vi "Dial Station Modem.vi"(8 "error in (no error)":errorcluster, 11 "Data Cluster in":T1={"Data Display"="", "FP Control Refs"={"Connect to Station Ref"=refnum, "Download Ref"=refnum, "Exit Button Ref"=refnum, "Start Date Refnum"=refnum, "End Date Refnum"=refnum, "Path"=refnum, "COM Port"="", "IP or Phone Ref"=refnum, "TCPIP ID"=refnum, "Reboot Refnum"=refnum, "Datafile Refnum"=refnum}, "FP Indicator Refs"={"Connected Refnum"=refnum, "Data Display Ref"=refnum, "Station ID Ref"=refnum}, "User Events"={"Stop"=refnum, "Update Display"=refnum}, "Message Queues"={"UI"=refnum, "ACQUISITION"=refnum, "PROCESSING"=refnum, "LOGGING"=refnum}, "IS IP?"=FALSE, "Downloading?"=FALSE, "DCP Version"=enum."XPert2", "Processing Loop State"=enum."Get Station  ID", "Username"=refnum, "Password"=refnum}) -> (0 "error out (no error)":errorcluster, 3 "Data Cluster out":T1={"Data Display"="", "FP Control Refs"={"Connect to Station Ref"=refnum, "Download Ref"=refnum, "Exit Button Ref"=refnum, "Start Date Refnum"=refnum, "End Date Refnum"=refnum, "Path"=refnum, "COM Port"="", "IP or Phone Ref"=refnum, "TCPIP ID"=refnum, "Reboot Refnum"=refnum, "Datafile Refnum"=refnum}, "FP Indicator Refs"={"Connected Refnum"=refnum, "Data Display Ref"=refnum, "Station ID Ref"=refnum}, "User Events"={"Stop"=refnum, "Update Display"=refnum}, "Message Queues"={"UI"=refnum, "ACQUISITION"=refnum, "PROCESSING"=refnum, "LOGGING"=refnum}, "IS IP?"=FALSE, "Downloading?"=FALSE, "DCP Version"=enum."XPert2", "Processing Loop State"=enum."Get Station  ID", "Username"=refnum, "Password"=refnum})   [LabVIEW 2018]
uses:
  controls/GLDL UI Data.ctl
  controls/Disconnect Control.ctl
  controls/Download Control.ctl
  controls/Exit Control.ctl
  controls/Date Control.ctl
  controls/IP Phone Number Control.ctl
  controls/Reboot Control.ctl
  controls/Connected Indicator.ctl
  controls/Output Indicator.ctl
  controls/Station ID Indicator.ctl
  Message Queue/All Message Queues.ctl
  Message Queue/Message Cluster.ctl
  controls/Processing Loop State.ctl
  Message Queue/GLDL Message Queue.lvlib
types:
  T1 = typedef "GLDL UI Data.ctl" = cluster{"Data Display":string, "FP Control Refs":cluster{"Connect to Station Ref":refnum<vi>, "Download Ref":refnum<vi>, "Exit Button Ref":refnum<vi>, "Start Date Refnum":refnum<vi>, "End Date Refnum":refnum<vi>, "Path":refnum<vi>, "COM Port":refnum<visa-resource-name>, "IP or Phone Ref":refnum<vi>, "TCPIP ID":refnum<k5>, "Reboot Refnum":refnum<vi>, "Datafile Refnum":refnum<file>}, "FP Indicator Refs":cluster{"Connected Refnum":refnum<vi>, "Data Display Ref":refnum<vi>, "Station ID Ref":refnum<vi>}, "User Events":cluster{"Stop":refnum<user-event>, "Update Display":refnum<user-event>}, "Message Queues":T2, "IS IP?":bool, "Downloading?":bool, "DCP Version":enum16{"XPert", "XPert2"}, "Processing Loop State":T3, "Username":refnum<vi>, "Password":refnum<vi>}
  T2 = typedef "GLDL Message Queue.lvlib/All Message Queues.ctl" = cluster{"UI":refnum<queue>, "ACQUISITION":refnum<queue>, "PROCESSING":refnum<queue>, "LOGGING":refnum<queue>}
  T3 = typedef "Processing Loop State.ctl" = enum16{"Get Station  ID", "Change Directory SD Card", "Change Directory Storage Card", "Downloading", "Idle in DL Directory"}
  T4 = typedef "IP Phone Number Control.ctl" = string
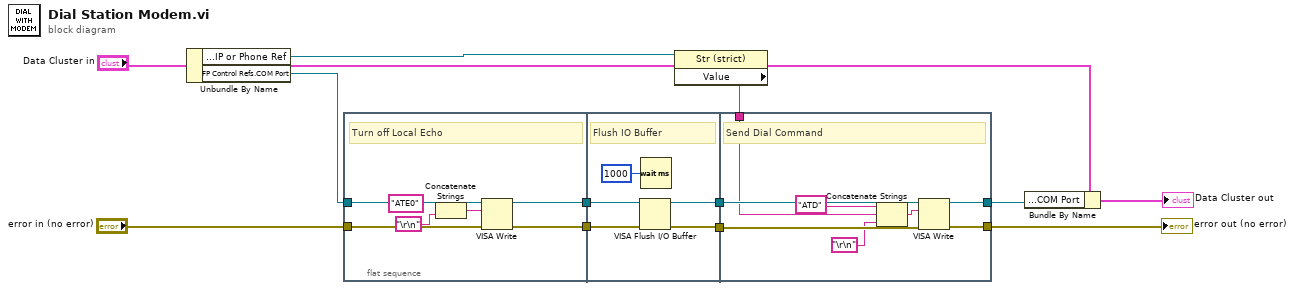
[diagram p0: block diagram]
diagram:
  n1 = Unbundle By Name("Data Cluster in") -> ("FP Control Refs.IP or Phone Ref"=w12:refnum<vi>, "FP Control Refs.COM Port"=w4:refnum<visa-resource-name>)
  n2 = flat-sequence {
    tunnel: "error in (no error)" -> [w18]
    tunnel: w4 -> [w15]
    tunnel: [w17] -> w10
    tunnel: [w16] -> w9
    tunnel: w10 -> [w23]
    tunnel: w9 -> [w24]
    tunnel: [w22] -> w8
    tunnel: [w21] -> w7
    tunnel: w8 -> [w32]
    tunnel: w7 -> [w31]
    tunnel: w6 -> [w27]
    tunnel: [w29] -> w5
    tunnel: [w26] -> w3
    frame #0 {
      # "Turn off Local Echo"
      n3 = Concatenate Strings("ATE0", "\r\n") -> (w19:string)
      n4 = VISA Write(VISA resource name=w15, write buffer=w19, error in (no error)=w18) -> (VISA resource name out=w16:refnum<visa-resource-name>, error out=w17:errorcluster)  [unwired: 1 out]
    }
    frame #1 {
      # "Flush IO Buffer"
      n5 = VISA Flush I/O Buffer(VISA resource name=w24, error in (no error)=w23) -> (VISA resource name out=w22:refnum<visa-resource-name>, error out=w21:errorcluster)  [unwired: 1 in]
      n6 = Wait (ms)(milliseconds to wait=u32 1000) -> ()  [unwired: 1 out]
    }
    frame #2 {
      # "Send Dial Command"
      n7 = Concatenate Strings("ATD", w27, "\r\n") -> (w28:string)
      n8 = VISA Write(VISA resource name=w32, write buffer=w28, error in (no error)=w31) -> (VISA resource name out=w26:refnum<visa-resource-name>, error out=w29:errorcluster)  [unwired: 1 out]
    }
  }
  n9 = property class="Str (strict)"(reference=w12) -> ("Value"=w6:T4)  [unwired: 1 in, 2 out]
  n10 = Bundle By Name(cluster="Data Cluster in", "FP Control Refs.COM Port"=w3) -> (→"Data Cluster out":T1)
  "error out (no error)" <- w5
